vi "Or77200_VisaRW.vi"(7 "Use LF-Cr":bool=TRUE, 8 "error in":errorcluster, 9 "ByteToRd":u32, 10 "Commande":string, 11 "Port":refnum<visa-resource-name>) -> (0 "error out":errorcluster {"code" format="%.0x"}, 1 "ByteRead":u32, 2 "Response":string, 3 "Port Out":refnum<visa-resource-name>)   [LabVIEW 2019]
uses:
  <vilib>/Instr/_visa.llb/VISA Configure Serial Port (Instr).vi
panel:
  out "ByteWr":u32
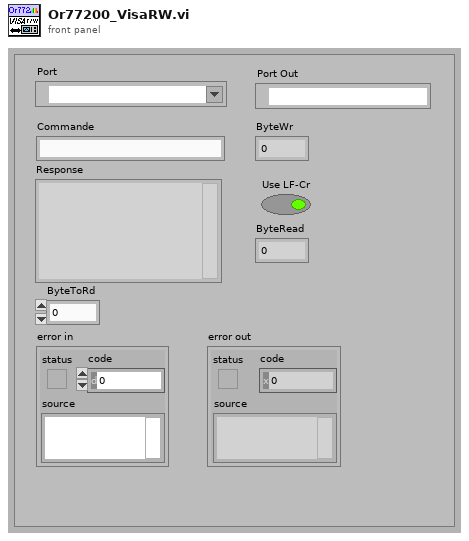
[diagram p1: front panel]
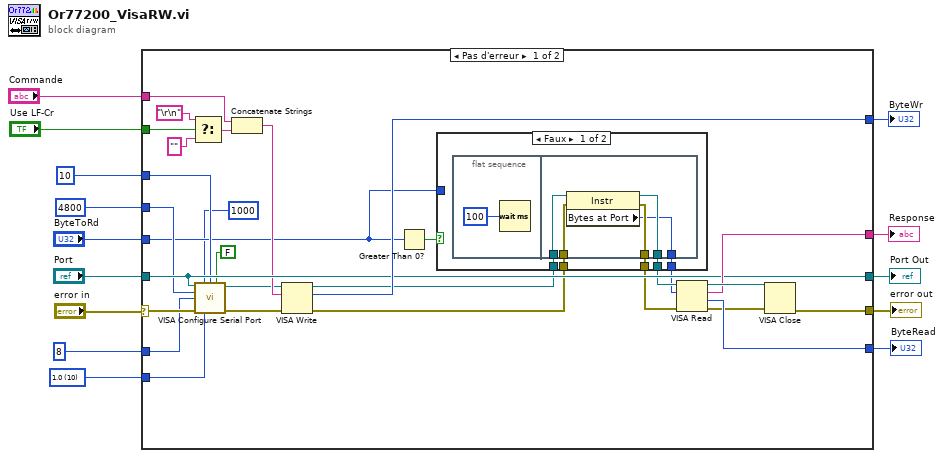
[diagram p0: block diagram]
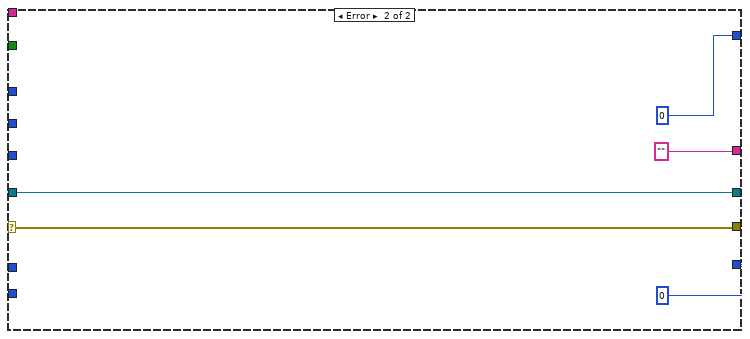
[diagram p3: hidden frame]
diagram:
  w1 = u16 10 items=["1.0"=10, "1.5"=15, "2.0"=20] ("stop bits (10: 1 bit)")
  n1 = case shown="Pas d'erreur" "error in" {
    selector: "error in" -> [w37 w59]
    tunnel: "Port" -> [w38 w62]
    tunnel: "Commande" -> [w31 _]
    tunnel: [w42 u32 0 ("return count")] -> w11
    tunnel: "ByteToRd" -> [w17 _]
    tunnel: [w41 "" ("read buffer")] -> w9
    tunnel: [w40 w59] -> w8
    tunnel: [w39 u32 0 ("return count")] -> w7
    tunnel: [w38 w62] -> w6
    tunnel: u16 8 ("Serial Settings:Data Bits") -> [w35 _]
    tunnel: u8 10 ("termination char\n(0xA = '\\n' = LF)") -> [w33 _]
    tunnel: u32 4800 ("Serial Settings:Baud Rate") -> [w32 _]
    tunnel: "Use LF-Cr" -> [w29 _]
    tunnel: w1 -> [w24 _]
    frame No Error {
      n2 = Select(t="\r\n", s=w29, f="" ("cas faux")) -> (s? t:f=w26:string)
      n3 = call-poly "VISA Configure Serial Port"("VISA resource name"=w38, "timeout (10sec)"=u32 1000, "termination char\n(0xA = '\\n' = LF)"=w33, "Enable Termination\nChar (T)"=FALSE ("Enable Termination\nChar (T)"), "baud rate (9600)"=w32, "data bits (8)"=w35, "error in (no error)"=w37, "stop bits (10: 1 bit)"=w24) -> ("VISA resource name out"=w25:refnum<visa-resource-name>, "error out"=w36:errorcluster)  [unwired: 6 in]
      n4 = Concatenate Strings(w31, w26) -> (w30:string)
      n5 = VISA Write(VISA resource name=w25, write buffer=w30, error in (no error)=w36) -> (VISA resource name out=w22:refnum<visa-resource-name>, return count=w42:u32, error out=w21:errorcluster)
      n6 = Greater Than 0?(x=w17) -> (x > 0?=w23:bool)
      n7 = case shown="Faux" w23 {
        tunnel: w22 -> [w48 w55]
        tunnel: w21 -> [w47 w56]
        tunnel: [w46 w56] -> w20
        tunnel: [w45 w55] -> w19
        tunnel: [w44 w57] -> w18
        tunnel: w17 -> [_ w57]
        frame False {
          n8 = flat-sequence {
            tunnel: w48 -> [w54]
            tunnel: w47 -> [w53]
            tunnel: [w52] -> w46
            tunnel: [w51] -> w45
            tunnel: [w50] -> w44
            frame #0 {
              n9 = Wait (ms)(milliseconds to wait=u32 100 ("attente (ms)")) -> ()  [unwired: 1 out]
            }
            frame #1 {
              n10 = property class="Instr"(reference=w54, error in=w53) -> (reference out=w51:refnum<visa-resource-name>, error out=w52:errorcluster, "Bytes at Port"=w50:u32)
            }
          }
        }
        frame True {
        }
      }
      n11 = VISA Read(VISA resource name=w19, byte count=w18, error in (no error)=w20) -> (VISA resource name out=w43:refnum<visa-resource-name>, read buffer=w41:string, return count=w39:u32, error out=w15:errorcluster)
      n12 = VISA Close(VISA resource name=w43, error in (no error)=w15) -> (error out=w40:errorcluster)
    }
    frame Error {
    }
  }
  "error out" <- w8
  "ByteWr" <- w11
  "Response" <- w9
  "ByteRead" <- w7
  "Port Out" <- w6
